vi "act-0021-3-cor.vi"() -> ()   [LabVIEW 2010]
uses:
  support/c_pi_wilson.ctl
  support/c_pi_penalite.ctl
  support/c_cout_choix_q.ctl
  support/lv_07.lvlib
panel:
  in  "Coût (e)":T1
  out "Coût (q=Qe)":T1
  in  "Pénalité (e)":T2
  in  "Pièce e":T3
  out "error out":errorcluster caption="err out"
  in  "err in":errorcluster
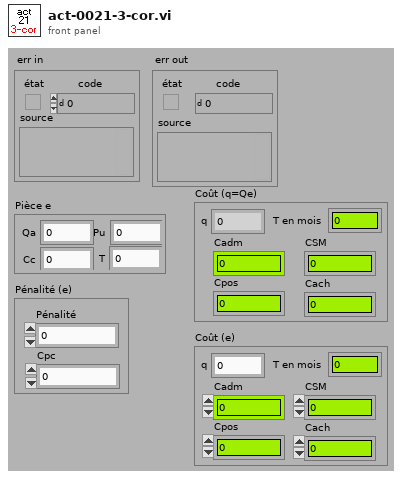
[diagram p1: front panel]
types:
  T1 = typedef "lv_07.lvlib/c_cout_choix_q.ctl" = cluster{"Cadm":dbl, "Cpos":dbl, "Cach":dbl, "CSM":dbl, "q":dbl, "T en mois":dbl}
  T2 = typedef "lv_07.lvlib/c_pi_penalite.ctl" = cluster{"Pénalité":dbl, "Cpc":dbl}
  T3 = typedef "lv_07.lvlib/c_pi_wilson.ctl" = cluster{"T":dbl, "Pu":dbl, "Qa":dbl, "Cc":dbl}
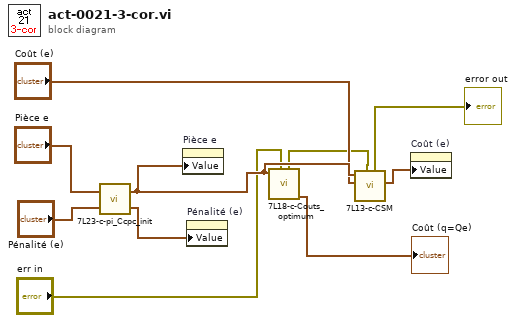
[diagram p0: block diagram]
diagram:
  n1 = call "7L23-c-pi_Ccpc_init.vi"("Pénalité (e)"="Pénalité (e)", "Pièce e"="Pièce e") -> ("Pénalité (s)"=w8:T2, "Pièce s"=w6:T3)
  n2 = property on="Pièce e" class="Clust (strict)"("Value"=w6) -> ()  [unwired: 2 in, 2 out]
  n3 = property on="Pénalité (e)" class="Clust (strict)"("Value"=w8) -> ()  [unwired: 2 in, 2 out]
  n4 = call "7L18-c-Couts_optimum.vi"("error in"="err in", "Pièce"=w6) -> ("Coût (q=Qe)"=→"Coût (q=Qe)":T1, "error out"=w3:errorcluster)  [unwired: 5 in, 1 out]
  n5 = call "7L13-c-CSM.vi"("err in"=w3, "Coût (e)"="Coût (e)", "Pièce (e)"=w6) -> ("Coût (s)"=w4:T1, "err out"=→"error out":errorcluster)  [unwired: 5 in]
  n6 = property on="Coût (e)" class="Clust (strict)"("Value"=w4) -> ()  [unwired: 2 in, 2 out]
